vi "Teleop.vi"(10 "Match Info":T1={"Autonomous Elapsed Seconds"=0.0, "TeleOp Elapsed Seconds"=0.0, "Disabled Elapsed Seconds"=0.0, "Visited Autonomous"=FALSE, "Visited TeleOp"=FALSE, "Visited Disabled"=FALSE, "Autonomous Settings"={"Autonomous Style"=enum."Independent", "VI Refnum"=refnum}}, 11 "Call Context":T2) -> ()   [LabVIEW 2013]
doc: "This VI is called for each TeleOp packet received from the DS where the robot is not disabled. It is often used to read from the joysticks and update I/O or to update setpoints for timed control loops. It should complete and return within 20 milliseconds or it may miss DS packets."
uses:
  <vilib>/Rock Robotics/WPI/DriverStation/WPI_DriverStationDerivedRobotMode.ctl
  <vilib>/Rock Robotics/WPI/DriverStation/WPI_DriverStationMatch Info.ctl
  RefnameEnum.ctl
  Robot Global Data.vi
  <vilib>/Rock Robotics/WPI/Joystick/WPI_JoystickGetSetRefNum.vi
  State_Machine_Enum.ctl
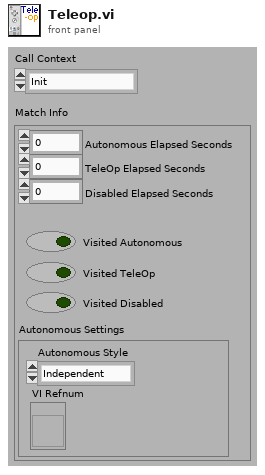
[diagram p1: front panel]
types:
  T1 = typedef "WPI_DriverStationMatch Info.ctl" = cluster{"Autonomous Elapsed Seconds":dbl, "TeleOp Elapsed Seconds":dbl, "Disabled Elapsed Seconds":dbl, "Visited Autonomous":bool, "Visited TeleOp":bool, "Visited Disabled":bool, "Autonomous Settings":cluster{"Autonomous Style":enum16{"Iterative", "Independent"}, "VI Refnum":refnum<vi>}}
  T2 = typedef "WPI_DriverStationDerivedRobotMode.ctl" = enum16{"Init", "Execute", "Stop"}
  T3 = typedef "State_Machine_Enum.ctl" = enum16{"Idle", "Start", "Do", "Stop", "Init"}
  T4 = typedef "RefnameEnum.ctl" = enum16{"FireLauncher", "Climber", "Shield", "TankDrive", "DriveEncoderL", "DriveEncoderR", "LauncherMotorRPM", "LauncherEncoderAnalog", "LauncherEncoderRPM", "ShooterLS", "DriveAlignLSLeft", "DriveAlignLSRight", "ClimbingLS", "LauncherEncoderAngle", "LauncherMotorAngle", "Gamepad1", "Gamepad2", "Compressor", "ClimbWeightSol3", "ClimbWeightSol4"}
  T5 = typedef "WPI_JoystickDevRef.ctl" = cluster{"Device":T6}
  T6 = typedef "WPI_JoystickDeviceEnum.ctl" = enum16{"USB 1", "USB 2", "USB 3", "USB 4", "Kinect 1", "Kinect 2"}
  T7 = typedef "WPI_JoystickButtonState.ctl" = cluster{"Button 1":bool, "Button 2":bool, "Button 3":bool, "Button 4":bool, "Button 5":bool, "Button 6":bool, "Button 7":bool, "Button 8":bool, "Button 9":bool, "Button 10":bool, "Button 11":bool, "Button 12":bool}
  T8 = cluster{"axis 1 (x)":dbl, "axis 2 (y)":dbl, "axis 3 (throttle)":dbl, "axis 4":dbl, "axis 5":dbl, "axis 6":dbl}
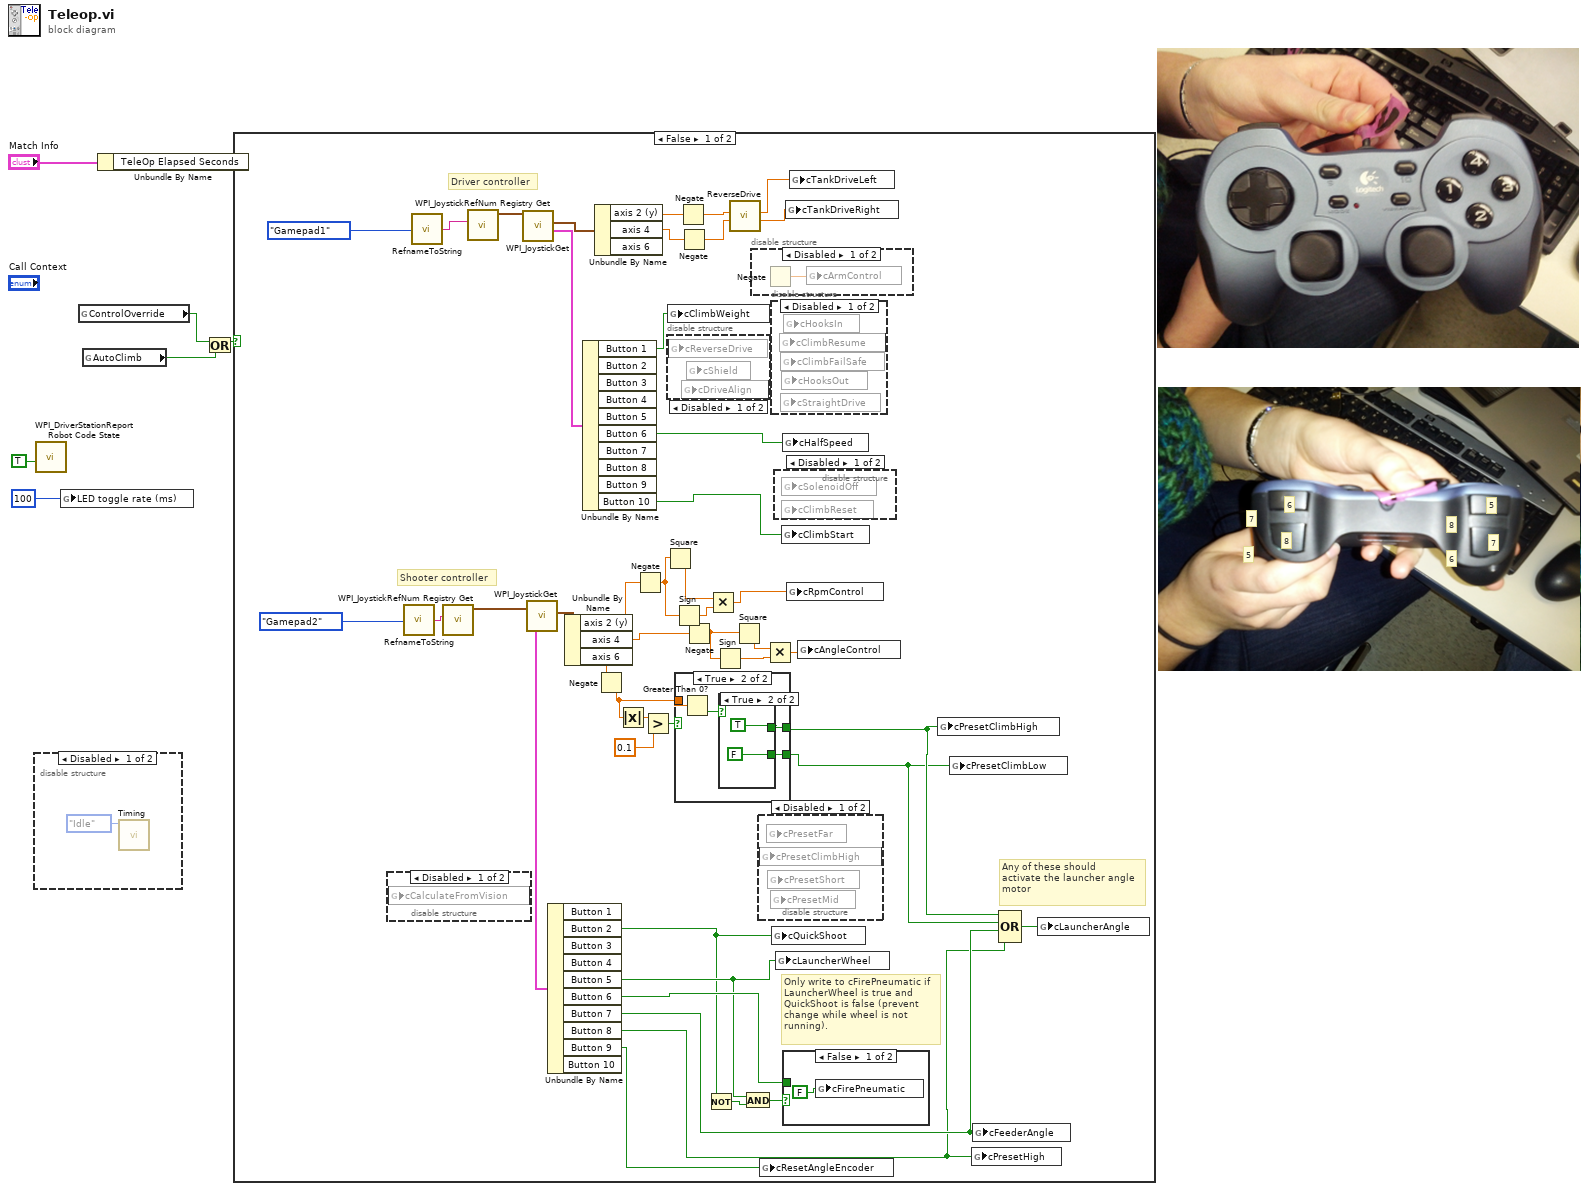
[diagram p0: block diagram]
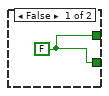
[diagram p5: hidden frame]
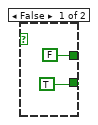
[diagram p6: hidden frame]
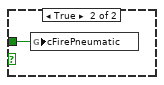
[diagram p7: hidden frame]
diagram:
  # "5"
  # "7"
  # "6"
  # "8"
  # "8"
  # "7"
  # "6"
  # "5"
  n1 = disable-structure shown="Disabled" {
    frame Disabled {
      n2 = call "Timing.vi"("State"=State_Machine_Enum."Idle") -> ()  [unwired: 9 in, 2 out]
    }
    frame Enabled {
    }
  }
  n3 = call <vilib>:"WPI_DriverStationReport Robot Code State.vi"("TeleOp"=TRUE ("Autonomous")) -> ()  [unwired: 10 in, 1 out]
  n4 = global write "Robot Global Data.vi" "LED toggle rate (ms)"(u32 100 ("LED ms toggle rate")) -> ()
  n5 = global read "Robot Global Data.vi" "ControlOverride"() -> (w3:bool)
  n6 = global read "Robot Global Data.vi" "AutoClimb"() -> (w1:bool)
  n7 = Unbundle By Name("Match Info") -> ()  [unwired: 1 out]
  n8 = Or(x=w3, y=w1) -> (x .or. y?=w2:bool)
  n9 = case shown="False" w2 {
    frame False {
      # "Any of these should\nactivate the launcher angle\nmotor"
      # "Only write to cFirePneumatic if LauncherWheel is true and QuickShoot is false (prevent change while wheel is not running)."
      # "Shooter controller"
      # "Driver controller"
      n10 = disable-structure shown="Disabled" {
        frame Disabled {
          n11 = global read "Robot Global Data.vi" "cCalculateFromVision"() -> ()  [unwired: 1 in]
        }
        frame Enabled {
        }
      }
      n12 = call "RefnameToString.vi"("Enum"=RefnameEnum."Gamepad2") -> ("Refname"=w23:string)
      n13 = call "RefnameToString.vi"("Enum"=RefnameEnum."Gamepad1") -> ("Refname"=w25:string)
      n14 = call <vilib>:"WPI_JoystickRefNum Registry Get.vi"("refnum name"=w23) -> ("JoystickDevRef"=w51:T5)  [unwired: 1 in, 9 out]
      n15 = call <vilib>:"WPI_JoystickRefNum Registry Get.vi"("refnum name"=w25) -> ("JoystickDevRef"=w52:T5)  [unwired: 1 in, 9 out]
      n16 = call <vilib>:"WPI_JoystickGet.vi"("JoystickDevRef"=w52) -> ("Buttons"=w48:T7, "Axes"=w50:T8)  [unwired: 4 in, 1 out]
      n17 = call <vilib>:"WPI_JoystickGet.vi"("JoystickDevRef"=w51) -> ("Buttons"=w46:T7, "Axes"=w47:T8)  [unwired: 4 in, 1 out]
      n18 = Unbundle By Name(w46) -> ("Button 2"=w15:bool, "Button 5"=w16:bool, "Button 6"=w45:bool, "Button 7"=w10:bool, "Button 8"=w9:bool, "Button 9"=w27:bool)  [unwired: 4 out]
      n19 = Unbundle By Name(w47) -> ("axis 2 (y)"=w42:dbl, "axis 4"=w40:dbl, "axis 6"=w22:dbl)
      n20 = Unbundle By Name(w48) -> ("Button 1"=w18:bool, "Button 6"=w37:bool, "Button 10"=w38:bool)  [unwired: 7 out]
      n21 = Unbundle By Name(w50) -> ("axis 2 (y)"=w49:dbl, "axis 4"=w31:dbl)  [unwired: 1 out]
      n22 = Negate(x=w22) -> (-x=w17:dbl)
      n23 = Absolute Value(x=w17) -> (abs(x)=w21:dbl)
      n24 = Negate(x=w42) -> (-x=w34:dbl)
      n25 = Greater?(x=w21, y=0.1) -> (0:w20:bool)
      n26 = Square(x=w34) -> (x^2=w44:dbl)
      n27 = global write "Robot Global Data.vi" "cClimbWeight"(w18) -> ()
      n28 = disable-structure shown="Disabled" {
        frame Disabled {
          n29 = global read "Robot Global Data.vi" "cReverseDrive"() -> ()  [unwired: 1 in]
          n30 = global read "Robot Global Data.vi" "cDriveAlign"() -> ()  [unwired: 1 in]
          n31 = global read "Robot Global Data.vi" "cShield"() -> ()  [unwired: 1 in]
        }
        frame Enabled {
        }
      }
      n32 = Sign(1:w34) -> (0:w43:dbl)
      n33 = case shown="True" w20 {
        tunnel: w17 -> [_ w56]
        tunnel: [w53 w55] -> w12
        tunnel: [w53 w54] -> w11
        frame False {
          w53 = FALSE
        }
        frame True {
          n34 = Greater Than 0?(x=w56) -> (x > 0?=w57:bool)
          n35 = case shown="True" w57 {
            tunnel: [FALSE TRUE] -> w55
            tunnel: [TRUE FALSE] -> w54
            frame False {
            }
            frame True {
            }
          }
        }
      }
      n36 = Negate(x=w49) -> (-x=w32:dbl)
      n37 = Negate(x=w31) -> (-x=w30:dbl)
      n38 = Negate(x=w40) -> (-x=w33:dbl)
      n39 = Not(x=w15) -> (.not. x?=w14:bool)
      n40 = Multiply(x=w44, y=w43) -> (x*y=w36:dbl)
      n41 = Sign(1:w33) -> (0:w41:dbl)
      n42 = call "ReverseDrive.vi"("InitLeft"=w32, "InitRight"=w30) -> ("Final Left"=w29:dbl, "FinalRight"=w28:dbl)  [unwired: 7 in]
      n43 = Square(x=w33) -> (x^2=w39:dbl)
      n44 = And(x=w16, y=w14) -> (x .and. y?=w13:bool)
      n45 = disable-structure shown="Disabled" {
        frame Disabled {
          n46 = Negate() -> (-x=w64:dbl)  [unwired: 1 in]
          n47 = global write "Robot Global Data.vi" "cArmControl"(w64) -> ()
        }
        frame Enabled {
        }
      }
      n48 = disable-structure shown="Disabled" {
        frame Disabled {
          n49 = global read "Robot Global Data.vi" "cPresetClimbHigh"() -> ()  [unwired: 1 in]
          n50 = global read "Robot Global Data.vi" "cPresetFar"() -> ()  [unwired: 1 in]
          n51 = global read "Robot Global Data.vi" "cPresetShort"() -> ()  [unwired: 1 in]
          n52 = global read "Robot Global Data.vi" "cPresetMid"() -> ()  [unwired: 1 in]
        }
        frame Enabled {
        }
      }
      n53 = global write "Robot Global Data.vi" "cResetAngleEncoder"(w27) -> ()
      n54 = Multiply(x=w39, y=w41) -> (x*y=w35:dbl)
      n55 = disable-structure shown="Disabled" {
        frame Disabled {
          n56 = global read "Robot Global Data.vi" "cClimbResume"() -> ()  [unwired: 1 in]
          n57 = global read "Robot Global Data.vi" "cClimbFailSafe"() -> ()  [unwired: 1 in]
          n58 = global read "Robot Global Data.vi" "cStraightDrive"() -> ()  [unwired: 1 in]
          n59 = global read "Robot Global Data.vi" "cHooksOut"() -> ()  [unwired: 1 in]
          n60 = global read "Robot Global Data.vi" "cHooksIn"() -> ()  [unwired: 1 in]
        }
        frame Enabled {
        }
      }
      n61 = global write "Robot Global Data.vi" "cQuickShoot"(w15) -> ()
      n62 = disable-structure shown="Disabled" {
        frame Disabled {
          n63 = global read "Robot Global Data.vi" "cSolenoidOff"() -> ()  [unwired: 1 in]
          n64 = global read "Robot Global Data.vi" "cClimbReset"() -> ()  [unwired: 1 in]
        }
        frame Enabled {
        }
      }
      n65 = global write "Robot Global Data.vi" "cLauncherWheel"(w16) -> ()
      n66 = global write "Robot Global Data.vi" "cClimbStart"(w38) -> ()
      n67 = global write "Robot Global Data.vi" "cHalfSpeed"(w37) -> ()
      n68 = case shown="False" w13 {
        tunnel: w45 -> [_ w63]
        frame False {
          n69 = global write "Robot Global Data.vi" "cFirePneumatic"(FALSE) -> ()
        }
        frame True {
          n70 = global write "Robot Global Data.vi" "cFirePneumatic"(w63) -> ()
        }
      }
      n71 = global write "Robot Global Data.vi" "cTankDriveRight"(w28) -> ()
      n72 = global write "Robot Global Data.vi" "cRpmControl"(w36) -> ()
      n73 = global write "Robot Global Data.vi" "cTankDriveLeft"(w29) -> ()
      n74 = global write "Robot Global Data.vi" "cAngleControl"(w35) -> ()
      n75 = global write "Robot Global Data.vi" "cPresetClimbHigh"(w12) -> ()
      n76 = global write "Robot Global Data.vi" "cPresetClimbLow"(w11) -> ()
      n77 = global write "Robot Global Data.vi" "cPresetHigh"(w9) -> ()
      n78 = global write "Robot Global Data.vi" "cFeederAngle"(w10) -> ()
      n79 = Compound Arithmetic op=OR(w12, w11, w10, w9) -> (w8:bool)
      n80 = global write "Robot Global Data.vi" "cLauncherAngle"(w8) -> ()
    }
    frame True {
    }
  }
